vi "APDcount_view.vi"() -> ()   [LabVIEW 2020]
panel:
  out "x-y":dbl
  in  "Path 2":path=path "I:/Trace/Trace CH2.tdms"
  in  "Path":path=path "I:/Trace/Trace CH1.tdms"
  out "Waveform Chart 2":dbl(graph)=116950.0
  out "Waveform Chart":dbl(graph)=116950.0
  out "channel2 rate 2":dbl format="%#.10g"
  out "channel1 rate":dbl format="%#.10g"
  in  "stop":bool
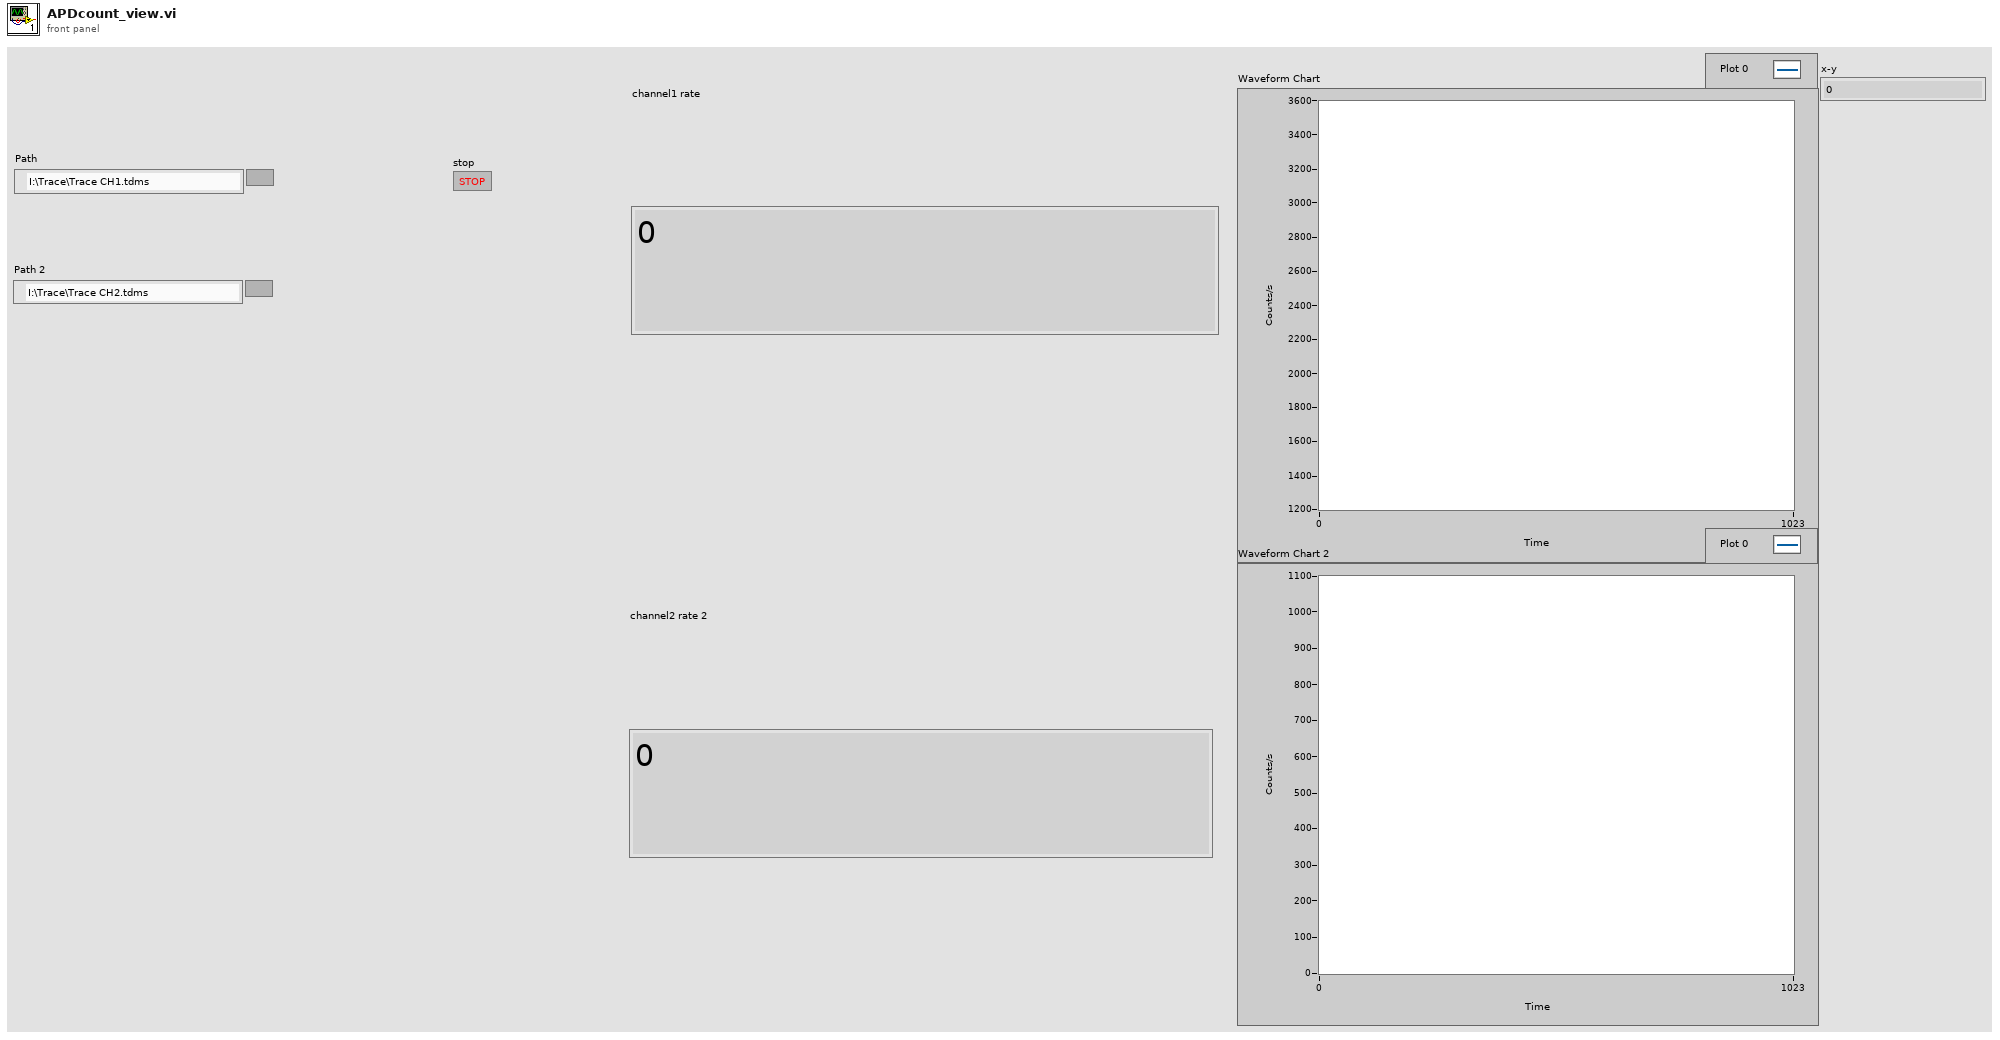
[diagram p1: front panel]
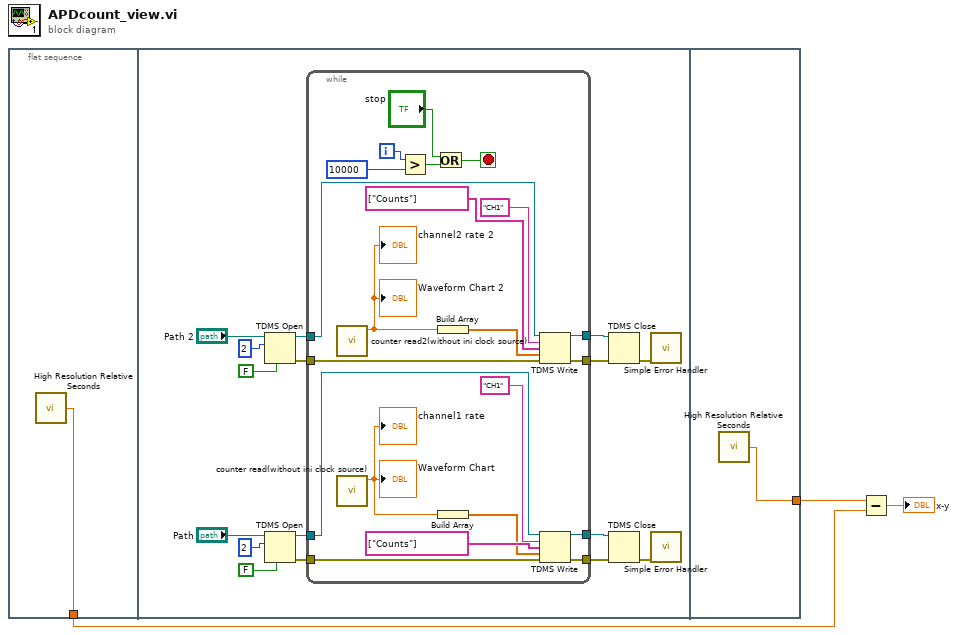
[diagram p0: block diagram]
diagram:
  n1 = flat-sequence {
    tunnel: [w4] -> w2
    tunnel: [w42] -> w3
    frame #0 {
      n2 = call <vilib>:"High Resolution Relative Seconds.vi"() -> ("relative seconds"=w4:dbl)
    }
    frame #1 {
      n3 = TDMS Open(6:FALSE ("disable buffering (T)"), 10:2, 11:"Path 2") -> (0:w6:errorcluster, 3:w5:refnum<k34>)  [unwired: 4 in]
      n4 = TDMS Open(6:FALSE ("disable buffering (T)"), 10:2, 11:"Path") -> (0:w10:errorcluster, 3:w14:refnum<k34>)  [unwired: 4 in]
      n5 = while {
        tunnel: w14 -> [w41]
        tunnel: [w36] -> w12
        tunnel: [w35] -> w11
        tunnel: w10 -> [w34]
        tunnel: [w32] -> w8
        tunnel: [w31] -> w7
        tunnel: w6 -> [w22]
        tunnel: w5 -> [w21]
        i -> [w27]
        stop <- w24 stop-if-true
        n6 = call "counter read2(without ini clock source).vi"() -> ("counter rate"=w29:dbl)  [unwired: 11 in]
        "channel2 rate 2" <- w29
        "Waveform Chart 2" <- w29
        n7 = call "counter read(without ini clock source).vi"() -> ("counter rate"=w38:dbl)  [unwired: 11 in]
        "channel1 rate" <- w38
        "Waveform Chart" <- w38
        n8 = Greater?(x=w27, y=10000) -> (0:w23:bool)
        n9 = Or(x="stop", y=w23) -> (x .or. y?=w24:bool)
        n10 = Build Array(w29) -> (w28:dbl[])
        n11 = Build Array(w38) -> (w37:dbl[])
        n12 = TDMS Write(0:w21, 5:"CH1" ("group name in (Untitled)"), 7:string[] ["Counts"] ("channel name(s) in (Untitled)"), 9:w28, 11:w22) -> (4:w32:refnum<k34>, 15:w31:errorcluster)  [unwired: 1 in, 2 out]
        n13 = TDMS Write(0:w41, 5:"CH1" ("group name in (Untitled)"), 7:string[] ["Counts"] ("channel name(s) in (Untitled)"), 9:w37, 11:w34) -> (4:w36:refnum<k34>, 15:w35:errorcluster)  [unwired: 1 in, 2 out]
      }
      n14 = TDMS Close(8:w7, 11:w8) -> (0:w9:errorcluster)  [unwired: 1 out]
      n15 = TDMS Close(8:w11, 11:w12) -> (0:w13:errorcluster)  [unwired: 1 out]
      n16 = call <vilib>:"Simple Error Handler.vi"("error in (no error)"=w9) -> ()  [unwired: 1 in, 8 out]
      n17 = call <vilib>:"Simple Error Handler.vi"("error in (no error)"=w13) -> ()  [unwired: 1 in, 8 out]
    }
    frame #2 {
      n18 = call <vilib>:"High Resolution Relative Seconds.vi"() -> ("relative seconds"=w42:dbl)
    }
  }
  n19 = Subtract(x=w3, y=w2) -> (x-y=→"x-y":dbl)
